vi "Send_Bash_Command.vi"(0 "working directory":path=path "/home/watchman/Documents/HV_Automation/CAENHV-master_2.0.1/Bash Script", 3 "Bash script":string="bash wavedump_bash.sh") -> (7 "Command Line Output":string, 8 "Over Temperature":bool, 9 "Event Build Error":bool, 10 "Error":string="LOL\n")   [LabVIEW 2018]
panel:
  out "offset of match 2":i32
  out "offset of match":i32
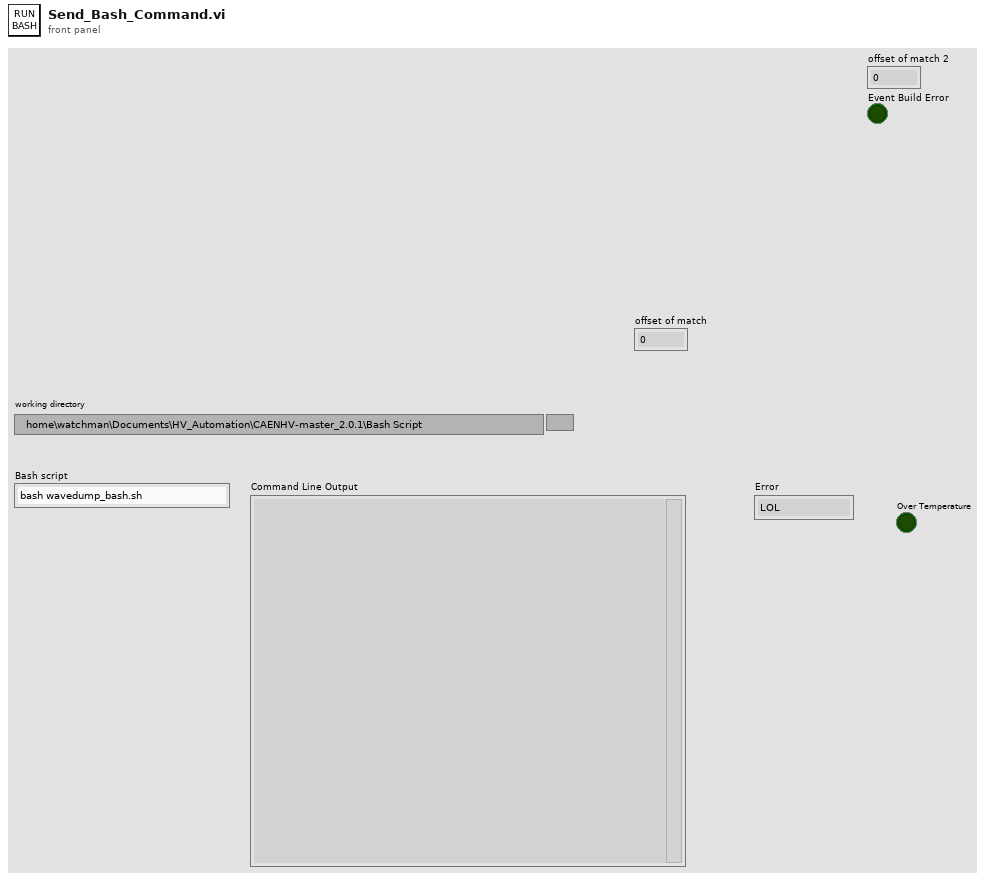
[diagram p1: front panel]
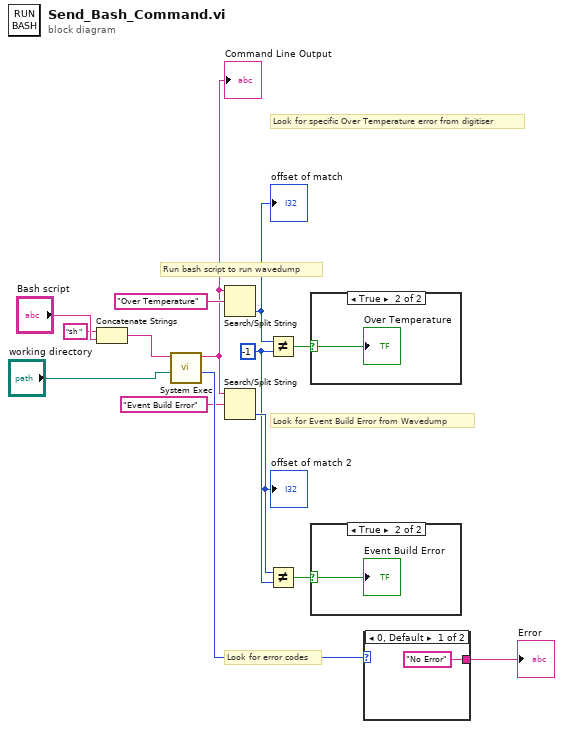
[diagram p0: block diagram]
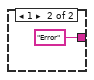
[diagram p4: hidden frame]
diagram:
  w4 = -1 ("y")
  # "Look for Event Build Error from Wavedump"
  # "Look for specific Over Temperature error from digitiser"
  # "Look for error codes"
  # "Run bash script to run wavedump"
  n1 = Concatenate Strings("sh " ("string"), "Bash script") -> (w1:string)
  n2 = call <vilib>:"System Exec.vi"("working directory"="working directory", "command line"=w1) -> ("return code"=w13:i32, "standard output"=w8:string)  [unwired: 6 in, 2 out]
  "Command Line Output" <- w8
  n3 = Search/Split String(string=w8, search string/char (-)="Over Temperature") -> (offset of match=w11:i32)  [unwired: 1 in, 2 out]
  "offset of match" <- w11
  n4 = Search/Split String(string=w8, search string/char (-)="Event Build Error") -> (offset of match=w6:i32)  [unwired: 1 in, 2 out]
  "offset of match 2" <- w6
  n5 = Not Equal?(x=w11, y=w4) -> (x != y?=w10:bool)
  n6 = Not Equal?(x=w6, y=w4) -> (x != y?=w5:bool)
  n7 = case shown="True" w10 {
    selector: w10 -> [_ w15]
    frame False {
    }
    frame True {
      "Over Temperature" <- w15
    }
  }
  n8 = case shown="True" w5 {
    selector: w5 -> [_ w16]
    frame False {
    }
    frame True {
      "Event Build Error" <- w16
    }
  }
  n9 = case shown="0, Default" w13 {
    tunnel: ["No Error" "Error"] -> w14
    frame 0, Default {
    }
    frame 1 {
    }
  }
  "Error" <- w14
